vi "Common_GetMilliSeconds.vi"(5 "error in (no error)":errorcluster) -> (17 "msValue":u32, 19 "error out":errorcluster)   [LabVIEW 2014]
doc: "Returns the value of the millisecond timer. The base reference time (millisecond zero) is undefined; that is, you cannot convert millisecond timer value to a real-world time or date. Be careful when you use this function in comparisons, because the value of the millisecond timer wraps from 2ˆ32-1 to 0."
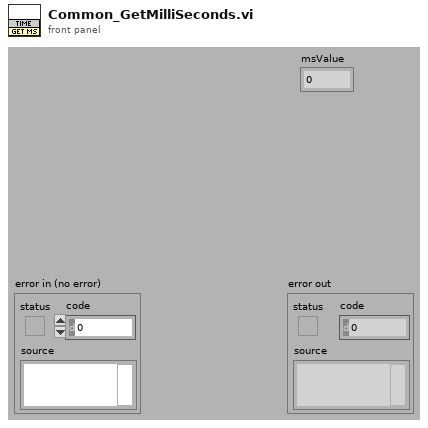
[diagram p1: front panel]
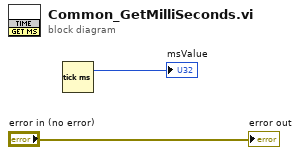
[diagram p0: block diagram]
diagram:
  n1 = Tick Count (ms)() -> (millisecond timer value=→"msValue":u32)
  "error out" <- "error in (no error)"
